vi "audioGen.vi"(6 "stop":bool, 8 "Frequency":dbl=500.0 format="%0.2p", 11 "Time Target (s)":dbl=1.0) -> (7 "stop 2":refnum<vi>)   [LabVIEW 2010]
uses:
  <vilib>/sound2/lvsound2.llb/Sampling Mode.ctl
  <vilib>/sound2/lvsound2.llb/Sound Data Format.ctl
  <vilib>/sound2/lvsound2.llb/Sound Output Write (DBL Single).vi
  <vilib>/measure/NI_MABase.lvlib
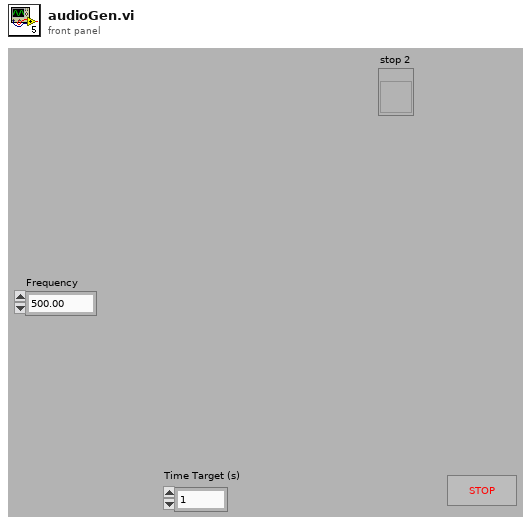
[diagram p1: front panel]
types:
  T1 = typedef "Sound Data Format.ctl" = cluster{"sample rate (S/s)":dbl, "number of channels":i32, "bits per sample":i32}
  T2 = typedef "Sampling Mode.ctl" = i32
  T3 = typedef "Sound Output Task ID.ctl" = u32
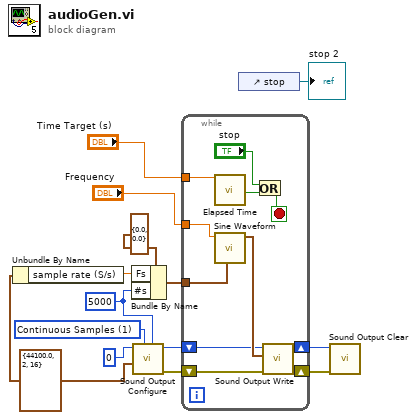
[diagram p0: block diagram]
diagram:
  w7 = 5000 ("Number of Samples/ch")
  w4 = T1 {"sample rate (S/s)"=44100.0, "number of channels"=2, "bits per sample"=16} ("Sound Format")
  w9 = T2 1 items=["Finite Samples", "Continuous Samples"] ("sample mode")
  n1 = Unbundle By Name(w4) -> ("sample rate (S/s)"=w5:dbl)
  n2 = Bundle By Name(cluster=cluster{"Fs":dbl, "#s":dbl} {"Fs"=0.0, "#s"=0.0} ("sampling info"), "Fs"=w5, "#s"=w7) -> (w6:cluster{"Fs":dbl, "#s":dbl})
  n3 = call <vilib>:"Sound Output Configure.vi"("number of samples/ch"=w7, "sample mode"=w9, "sound format"=w4, "device ID"=u32 0 ("Device ID")) -> ("error out"=w14:errorcluster, "task ID"=w13:T3)  [unwired: 6 in]
  n4 = while {
    shift-right: [w24] -> w12
    shift-left: w14 -> [w17]
    shift-right: [w25] -> w11
    shift-left: w13 -> [w18]
    tunnel: w6 -> [w23]
    tunnel: "Time Target (s)" -> [w20]
    tunnel: "Frequency" -> [w15]
    stop <- w19 stop-if-true
    n5 = call "Elapsed Time"("Time Target (s)"=w20) -> ("Time has Elapsed"=w21:bool)  [unwired: 11 in, 7 out]
    n6 = call <vilib>:"Sine Waveform.vi"("sampling info"=w23, "frequency"=w15) -> ("signal out"=w22:waveform(dbl))  [unwired: 8 in, 1 out]
    n7 = Or(x="stop", y=w21) -> (x .or. y?=w19:bool)
    n8 = call-poly <vilib>:"Sound Output Write.vi"("error in (no error)"=w17, "data"=w22, "task ID"=w18) -> ("error out"=w24:errorcluster, "task ID out"=w25:T3)  [unwired: 7 in]
  }
  n9 = control-ref of="stop"() -> (→"stop 2":refnum<vi>)
  n10 = call <vilib>:"Sound Output Clear.vi"("error in (no error)"=w12, "task ID"=w11) -> ()  [unwired: 9 in, 1 out]
